vi "Run Offline Judge.vi"() -> ()   [LabVIEW 2014]
uses:
  Main Contest/Problem.ctl
panel:
  in  "TestCases Folder":path=path "C:/Users/Justin/Desktop/LabVIEW-Rank/Offline Judge/TestCases"
  in  "Problem":T1
  out "Accept?":bool
  # "You MUST have the path to the TestCases Folder entered before any tests can be run"
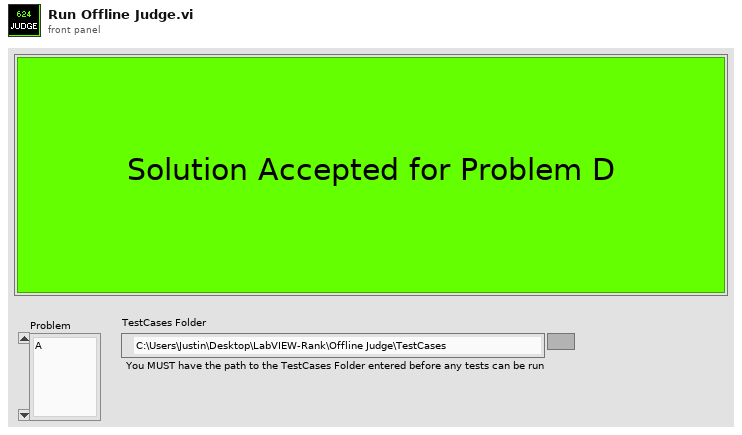
[diagram p1: front panel]
types:
  T1 = typedef "Problem.ctl" = enum16{"A", "B", "C", "D", "E"}
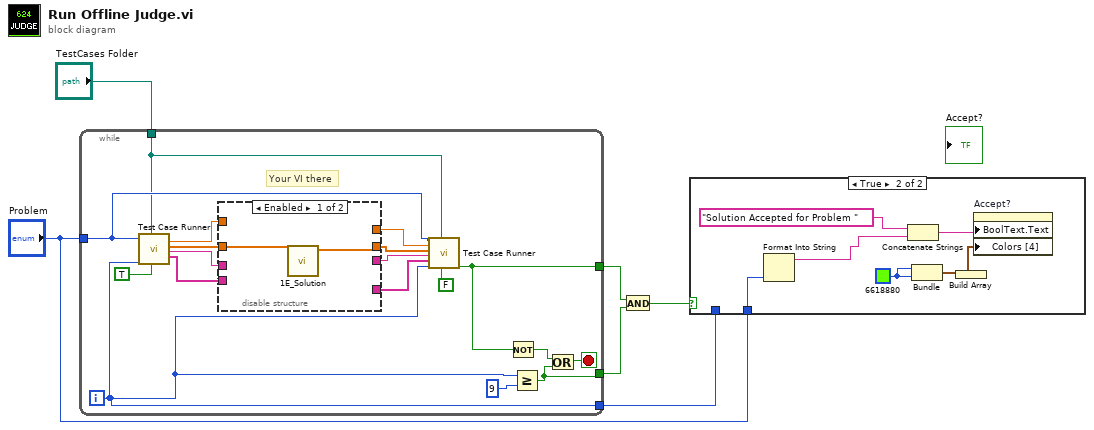
[diagram p0: block diagram]
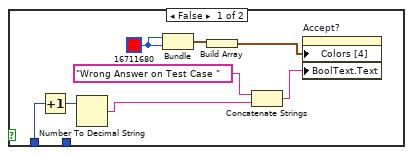
[diagram p2: hidden frame]
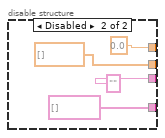
[diagram p3: hidden frame]
diagram:
  n1 = while {
    tunnel: "Problem" -> [w19]
    tunnel: [w21] -> w5
    tunnel: [w17] -> w4
    tunnel: [w8] -> w6
    tunnel: "TestCases Folder" -> [w7]
    i -> [w17]
    stop <- w18 stop-if-true
    # "Your VI there"
    n2 = call "Test Case Runner.vi"("Problem"=w19, "Iterator"=w17, "TestCases Folder"=w7, "Send Input?"=TRUE ("Input")) -> ("Numeric"=w16:dbl, "Numeric Array"=w15:dbl[], "String"=w14:string, "String Array"=w13:string[])  [unwired: 11 in, 1 out]
    n3 = disable-structure shown="Enabled" {
      disable-tunnel: w16 -> [_ _]
      disable-tunnel: w15 -> [w26 _]
      disable-tunnel: w14 -> [_ _]
      disable-tunnel: w13 -> [_ _]
      disable-tunnel: [_ 0.0 ("Numeric")] -> w12
      disable-tunnel: [w25 dbl[] [] ("Numeric Array")] -> w11
      disable-tunnel: [_ "" ("String")] -> w10
      disable-tunnel: [_ string[] [] ("String Array")] -> w9
      frame Enabled {
        n4 = call "1E_Solution.vi"("Array"=w26) -> ("Array 2"=w25:dbl[])  [unwired: 10 in]
      }
      frame Disabled {
      }
    }
    n5 = call "Test Case Runner.vi"("Problem"=w19, "Numeric 2"=w12, "Numeric Array 2"=w11, "String 2"=w10, "String Array 2"=w9, "Iterator"=w17, "TestCases Folder"=w7, "Send Input?"=FALSE) -> ("Accepted"=w8:bool)  [unwired: 7 in, 4 out]
    n6 = Not(x=w8) -> (.not. x?=w22:bool)
    n7 = Greater Or Equal?(x=w17, y=9) -> (x >= y?=w21:bool)
    n8 = Or(x=w22, y=w21) -> (x .or. y?=w18:bool)
  }
  n9 = And(x=w6, y=w5) -> (x .and. y?=w3:bool)
  n10 = case shown="True" w3 {
    tunnel: w4 -> [w32 _]
    tunnel: "Problem" -> [_ w41]
    frame False {
      w37 = u32 16711680
      n11 = Increment(x=w32) -> (x+1=w31:i32)
      n12 = Number To Decimal String(number=w31) -> (decimal integer string=w33:string)  [unwired: 1 in]
      n13 = Bundle(w37, w37) -> (w38:cluster{u32, u32})  [unwired: 1 in]
      n14 = Build Array(w38) -> (w36:cluster{u32, u32}[])
      n15 = Concatenate Strings("Wrong Answer on Test Case " ("Boolean Text.Text"), w33) -> (w34:string)
      n16 = property on="Accept?" class="Bool (strict)"("Colors [4]"=w36, "BoolText.Text"=w34) -> ()  [unwired: 2 in, 2 out]
    }
    frame True {
      w45 = u32 6618880
      n17 = Format Into String(w41) -> (resulting string=w42:string)  [unwired: 3 in, 1 out]
      n18 = Concatenate Strings("Solution Accepted for Problem " ("Boolean Text.Text"), w42) -> (w39:string)
      n19 = Bundle(w45, w45) -> (w44:cluster{u32, u32})  [unwired: 1 in]
      n20 = Build Array(w44) -> (w43:cluster{u32, u32}[])
      n21 = property on="Accept?" class="Bool (strict)"("BoolText.Text"=w39, "Colors [4]"=w43) -> ()  [unwired: 2 in, 2 out]
    }
  }
